vi "NoiseOutput_PXI-7813R.vi"() -> ()   [LabVIEW 2012]
uses:
  <vilib>/Platform/TimedLoop/XDataNode/timing_clust.ctl
  <vilib>/Platform/TimedLoop/XDataNode/nitl_modes.ctl
  <vilib>/Platform/TimedLoop/XDataNode/wakeup.ctl
  <vilib>/rvi/Emulation/niFpgaSctlEmulationRegisterWithScheduler.vi
  <vilib>/rvi/Emulation/niFpgaSctlEmulationGlobalWrite.vi
  <vilib>/rvi/eio/common/nirviEmuTemplateMethod_errors.vi
  <vilib>/rvi/interface/RandomDataEmulation/nirviRandomDataFPGAFIFO.vi
  <vilib>/rvi/interface/RandomDataEmulation/niFpgaRandomDataHandleErrors.vi
  <vilib>/rvi/Emulation/niFpgaSctlEmulationScheduler.vi
  <vilib>/Platform/TimedLoop/XDataNode/XDataNode.xnode
  <vilib>/eio/EIONode/EIONode.xnode
  <vilib>/rvi/DataTransferAndStorage/Container/XNode/niFpgaContainer.xnode
  <vilib>/rvi/interface/RandomDataEmulation/nirviRandomDataFpgaReadWriteTemplate.vi
  <vilib>/Platform/TimedLoop/XDataNode/XDNodeRunTimeDep.lvlib
panel:
  out "Acquiring":bool
  out "ToHostCh2Overflow":bool
  out "ToHostCh1Overflow":bool
  in  "Quit":bool
  in  "Samples per pixel":u32
  in  "Samples per line":u32
  in  "Samples per frame":u32
  in  "Requested pixels":u32=100000
  in  "Acquire continuously":bool=TRUE
  in  "Acquire":bool
  in  "Wait for trigger":bool
  # "Acquisition control"
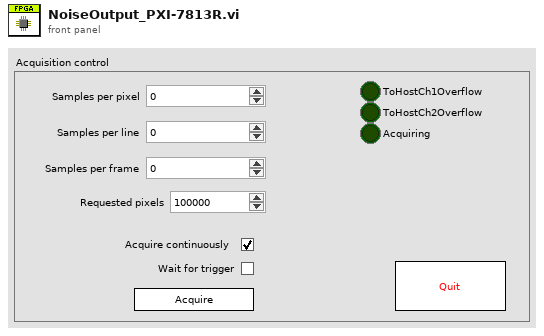
[diagram p1: front panel]
types:
  T1 = typedef "XDNodeRunTimeDep.lvlib/timing_clust.ctl" = cluster{"Expected End [f-1]":u64, "Actual End [f-1]":u64, "Finished Late? [f-1]":bool, "Expected End [i-1]":u64, "Actual End [i-1]":u64, "Finished Late? [i-1]":bool, "Expected Start [i]":u64, "Actual Start [i]":u64, "Expected Start [f]":u64, "Actual Start [f]":u64, "Source Name":string, "Structure Name":string, "Period":i64, "Deadline":i64, "Offset":i64, "Start":i64, "Priority":i32, "Timeout":i32, "Mode":T2, "Wakeup Reason":T3, "Error":errorcluster, "Source Type":string, "Secondary Source Type":string, "Global End Time":u64, "Global Start Time":u64, "Frame Duration":u64, "Iteration Duration":u64, "Assigned CPU":i32, "I/O Scan Engine Mode":u32}
  T2 = typedef "XDNodeRunTimeDep.lvlib/nitl_modes.ctl" = enum32{"No Change", "Process missed periods, maintain original phase", "Discard missed periods, maintain original phase", "Process missed periods, ignore original phase", "Discard missed periods, ignore original phase"}
  T3 = typedef "XDNodeRunTimeDep.lvlib/wakeup.ctl" = enum32{"Normal", "Aborted", "Asynchronous wakeup", "Timing source error", "Timed loop error", "Timeout"}
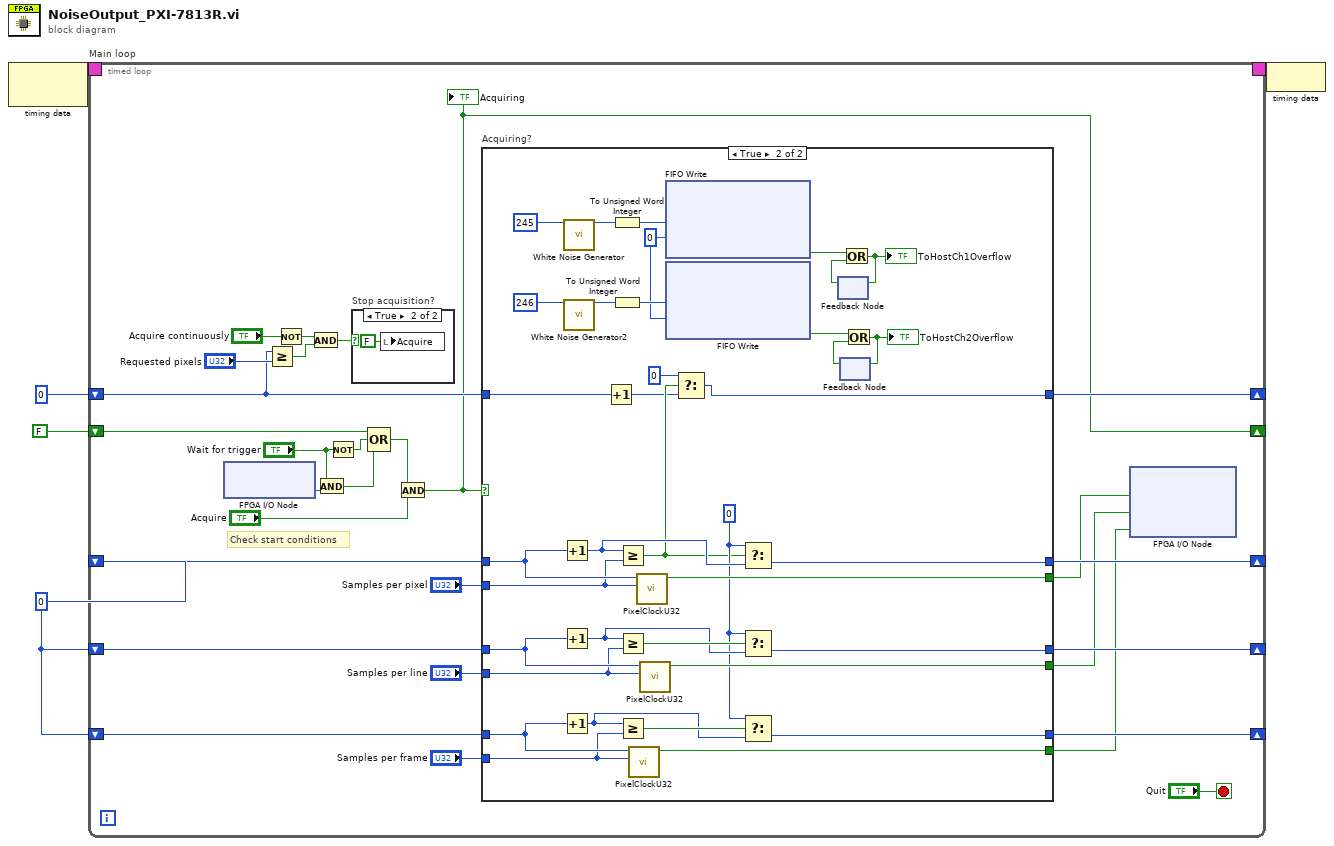
[diagram p0: block diagram]
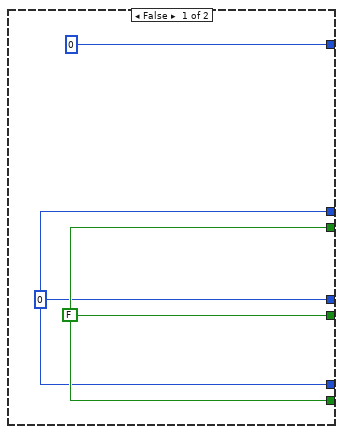
[diagram p3: hidden frame]
diagram:
  w3 = u32 0 ("Cycle counter out")
  n1 = node-c288() -> (w5:T1)  [unwired: 1 in]
  n2 = timed-loop "Main loop" {
    timing: w5 -> [_]
    timing-out: [_] -> w4
    shift-right: [w32] -> _
    shift-left: w3 -> [w31]
    shift-right: [w29] -> _
    shift-left: w3 -> [w28]
    shift-right: [w26] -> _
    shift-left: w3 -> [w25]
    shift-right: [w6] -> _
    shift-left: FALSE -> [w9]
    shift-right: [w7] -> _
    shift-left: u32 0 -> [w8]
    stop <- "Quit" stop-if-true
    # "Check start conditions"
    n3 = xnode "FPGA I/O Node"() -> ("TriggerIn"=w15:bool)  [unwired: 1 in, 1 out]
    n4 = Greater Or Equal?(x=w8, y="Requested pixels") -> (x >= y?=w17:bool)
    n5 = Not(x="Acquire continuously") -> (.not. x?=w18:bool)
    n6 = And(x=w18, y=w17) -> (x .and. y?=w16:bool)
    n7 = And(x="Wait for trigger", y=w15) -> (x .and. y?=w12:bool)
    n8 = Not(x="Wait for trigger") -> (.not. x?=w13:bool)
    n9 = case "Stop acquisition?" shown="True" w16 {
      frame False {
      }
      frame True {
        n10 = local write "Acquire"(FALSE ("Acquire")) -> ()
      }
    }
    n11 = Compound Arithmetic op=OR(w9, w13, w12) -> (w11:bool)
    n12 = And(x=w11, y="Acquire") -> (x .and. y?=w6:bool)
    "Acquiring" <- w6
    n13 = case "Acquiring?" shown="True" w6 {
      tunnel: [w36 w63] -> w32
      tunnel: w31 -> [_ w71]
      tunnel: "Samples per pixel" -> [_ w70]
      tunnel: [w36 w62] -> w29
      tunnel: w28 -> [_ w66]
      tunnel: "Samples per line" -> [_ w65]
      tunnel: [w36 w57] -> w26
      tunnel: w25 -> [_ w59]
      tunnel: "Samples per frame" -> [_ w58]
      tunnel: [w37 w72] -> w23
      tunnel: [w37 w64] -> w22
      tunnel: [w37 w56] -> w21
      tunnel: w8 -> [_ w52]
      tunnel: [u32 0 ("t") w50] -> w7
      frame False {
        w36 = u32 0 ("t")
        w37 = FALSE
      }
      frame True {
        w44 = 0 ("Timeout")
        w55 = u32 0 ("t")
        n14 = Increment(x=w71) -> (x+1=w69:u32)
        n15 = Increment(x=w66) -> (x+1=w67:u32)
        n16 = Increment(x=w59) -> (x+1=w60:u32)
        n17 = call "White Noise Generator"("seed"=u32 245) -> ("white noise out"=w48:i16)  [unwired: 14 in]
        n18 = call "White Noise Generator2"("seed"=u32 246) -> ("white noise out"=w46:i16)  [unwired: 14 in]
        n19 = Increment(x=w52) -> (x+1=w53:u32)
        n20 = To Unsigned Word Integer(number=w48) -> (unsigned 16bit integer=w47:u16)
        n21 = To Unsigned Word Integer(number=w46) -> (unsigned 16bit integer=w45:u16)
        n22 = Greater Or Equal?(x=w69, y=w70) -> (x >= y?=w54:bool)
        n23 = Greater Or Equal?(x=w67, y=w65) -> (x >= y?=w68:bool)
        n24 = Greater Or Equal?(x=w60, y=w58) -> (x >= y?=w61:bool)
        n25 = call "PixelClockU32.vi"("Samples per pixel"=w58, "Sample counter"=w59) -> ("Pixel clock"=w56:bool)  [unwired: 9 in]
        n26 = call "PixelClockU32.vi"("Samples per pixel"=w70, "Sample counter"=w71) -> ("Pixel clock"=w72:bool)  [unwired: 9 in]
        n27 = call "PixelClockU32.vi"("Samples per pixel"=w65, "Sample counter"=w66) -> ("Pixel clock"=w64:bool)  [unwired: 9 in]
        n28 = xnode "FIFO Write"("Element"=w47, "Timeout"=w44) -> ("Timed Out?"=w42:bool)  [unwired: 1 in, 1 out]
        n29 = xnode "FIFO Write"("Element"=w45, "Timeout"=w44) -> ("Timed Out?"=w39:bool)  [unwired: 1 in, 1 out]
        n30 = Select(t=u32 0, s=w54, f=w53) -> (s? t:f=w50:u32)
        n31 = Select(t=w55, s=w54, f=w69) -> (s? t:f=w63:u32)
        n32 = Select(t=w55, s=w68, f=w67) -> (s? t:f=w62:u32)
        n33 = Select(t=w55, s=w61, f=w60) -> (s? t:f=w57:u32)
        n34 = feedback #1() -> (w41:bool)  [unwired: 1 in]
        n35 = feedback #2() -> (w38:bool)  [unwired: 1 in]
        n36 = Or(x=w42, y=w41) -> (x .or. y?=w43:bool)
        "ToHostCh1Overflow" <- w43
        n37 = feedback-in #1(w43) -> ()
        n38 = Or(x=w39, y=w38) -> (x .or. y?=w40:bool)
        "ToHostCh2Overflow" <- w40
        n39 = feedback-in #2(w40) -> ()
      }
    }
    n40 = xnode "FPGA I/O Node"("PixelClock"=w23, "LineClock"=w22, "FrameClock"=w21) -> ()  [unwired: 3 in, 3 out]
  }
  n41 = node-c288(w4) -> ()
